vi "Check Waveforms.vi"(6 "Order In":u16, 7 "Tab is on R?":bool, 8 "Error In (no Error) In":errorcluster, 10 "X/R In":refnum<vi>, 11 "Y/Theta In":refnum<vi>) -> (0 "Error Out":errorcluster, 1 "Y/Theta  Out":waveform(dbl), 3 "X/R  Out":waveform(dbl))   [LabVIEW 2012, in "Vector Function Generator.xctl"]
doc: "If both components are being varied at the same time, ensure that they have equal numbers of points"
uses:
  Vector Function Generator.xctl
  <userlib>/_LAVAcr/User_Interface/XControls/Waveform_XControl/Waveform Control.xctl
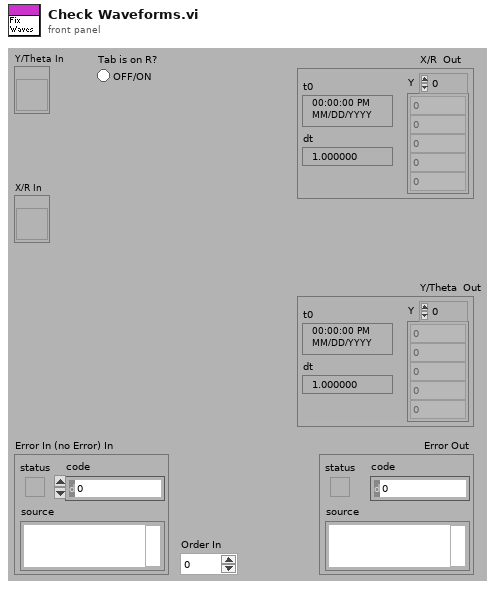
[diagram p1: front panel]
types:
  T1 = enum16{"R then Theta", "Theta then R", "R and Theta"}
  T2 = typedef "Waveform Control.xctl/FP Controls.ctl" = cluster{"Type":T3, "Periods":dbl, "Points":i32, "Offset":dbl, "Amplitdue":dbl, "Phase":dbl, "func":string}
  T3 = typedef "Waveform Control.xctl/Function Types.ctl" = enum16{"Level", "Sine", "Triangle", "Ramp", "Saw Tooth", "Square", "Function"}
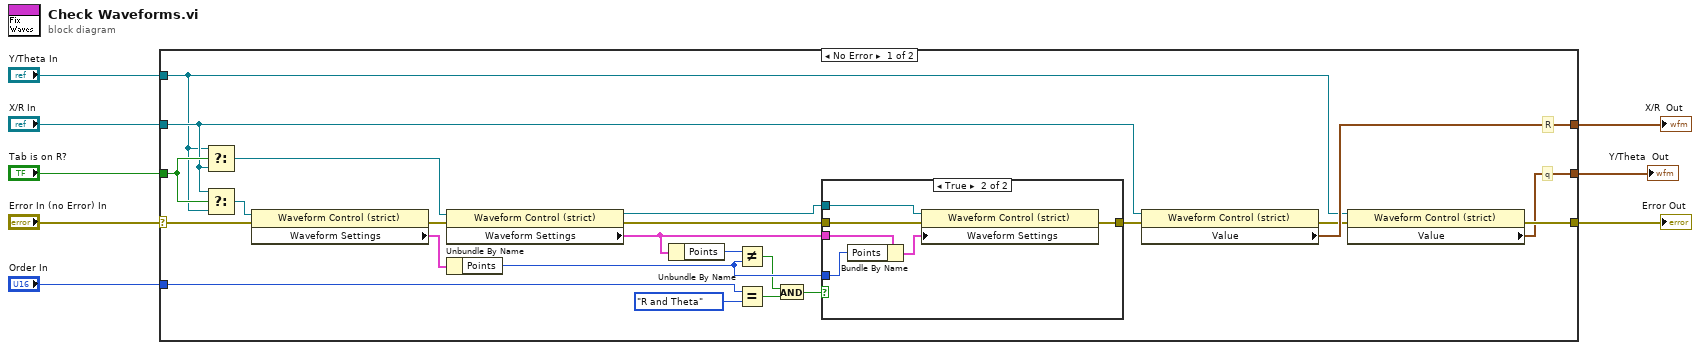
[diagram p0: block diagram]
diagram:
  n1 = case shown="No Error" "Error In (no Error) In" {
    selector: "Error In (no Error) In" -> [w30 w39]
    tunnel: [w31 w39] -> w8
    tunnel: [w29 _] -> w6
    tunnel: [w28 _] -> w5
    tunnel: "Order In" -> [w27 _]
    tunnel: "Tab is on R?" -> [w12 _]
    tunnel: "X/R In" -> [w11 _]
    tunnel: "Y/Theta In" -> [w10 _]
    frame No Error {
      # "q"
      # "R"
      n2 = Select(t=w10, s=w12, f=w11) -> (s? t:f=w13:refnum<vi>)
      n3 = Select(t=w11, s=w12, f=w10) -> (s? t:f=w9:refnum<vi>)
      n4 = property class="Waveform Control (strict)"(reference=w9, error in=w30) -> (error out=w20:errorcluster, "Waveform Settings"=w14:T2)  [unwired: 1 out]
      n5 = property class="Waveform Control (strict)"(reference=w13, error in=w20) -> (reference out=w18:refnum<vi>, error out=w21:errorcluster, "Waveform Settings"=w17:T2)
      n6 = Unbundle By Name(w14) -> ("Points"=w19:i32)
      n7 = Unbundle By Name(w17) -> ("Points"=w15:i32)
      n8 = Not Equal?(x=w15, y=w19) -> (x != y?=w16:bool)
      n9 = Equal?(x=w27, y=T1."R and Theta") -> (x = y?=w25:bool)
      n10 = And(x=w16, y=w25) -> (x .and. y?=w24:bool)
      n11 = case shown="True" w24 {
        tunnel: w17 -> [_ w38]
        tunnel: w18 -> [_ w36]
        tunnel: w19 -> [_ w35]
        tunnel: w21 -> [w32 w34]
        tunnel: [w32 w33] -> w23
        frame False {
        }
        frame True {
          n12 = Bundle By Name(cluster=w38, "Points"=w35) -> (w37:T2)
          n13 = property class="Waveform Control (strict)"(reference=w36, error in=w34, "Waveform Settings"=w37) -> (error out=w33:errorcluster)  [unwired: 1 out]
        }
      }
      n14 = property class="Waveform Control (strict)"(reference=w11, error in=w23) -> (error out=w22:errorcluster, "Value"=w28:waveform(dbl))  [unwired: 1 out]
      n15 = property class="Waveform Control (strict)"(reference=w10, error in=w22) -> (error out=w31:errorcluster, "Value"=w29:waveform(dbl))  [unwired: 1 out]
    }
    frame Error {
    }
  }
  "Error Out" <- w8
  "Y/Theta  Out" <- w6
  "X/R  Out" <- w5
